vi "Version From Tree.vi"(8 "error in":errorcluster, 11 "XML in":string) -> (0 "error out":errorcluster, 2 "Version":i32, 3 "XML out":string)   [LabVIEW 2020]
uses:
  <vilib>/addons/analyzer/_vianuishared.llb/VIAnUI CFG File Info Global.vi
  <vilib>/addons/analyzer/XML Parsing/NI_VIAn_XML Parsing.lvlib
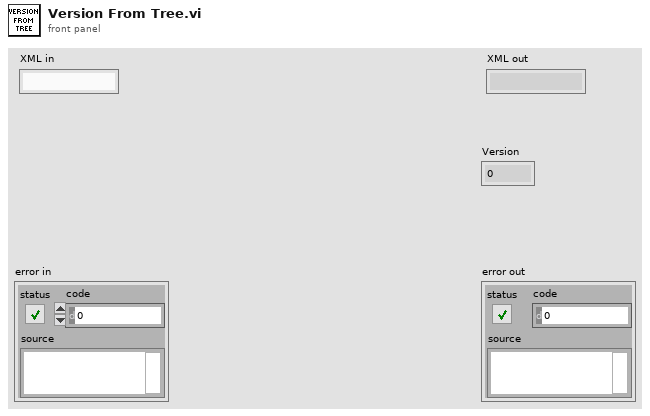
[diagram p1: front panel]
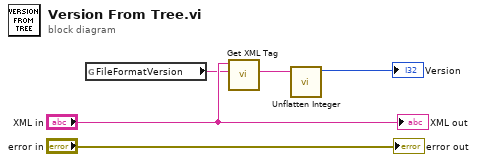
[diagram p0: block diagram]
diagram:
  n1 = global read "VIAnUI CFG File Info Global.vi" "FileFormatVersion"() -> (w3:string)
  n2 = call <vilib>:"Get XML Tag.vi"("Tag name"=w3, "XML String in"="XML in") -> ("Tag value"=w2:string)  [unwired: 5 in, 4 out]
  n3 = call <vilib>:"Unflatten Integer.vi"("Tag value"=w2) -> ("Numeric"=→"Version":i32)  [unwired: 10 in]
  "error out" <- "error in"
  "XML out" <- "XML in"
